vi "ErrorLog_ClearErrors.vi"(7 "Owner":string, 8 "error in (no error)":errorcluster, 11 "reference in":refnum<class "ErrorLog.lvclass">) -> (0 "error out":errorcluster, 3 "reference out":refnum<class "ErrorLog.lvclass">)   [LabVIEW 2014, in "ErrorLog.lvclass"]
uses:
  ErrorLog.lvclass
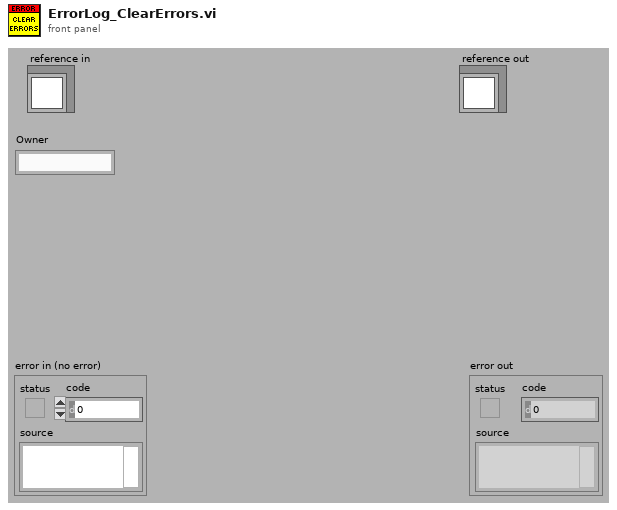
[diagram p1: front panel]
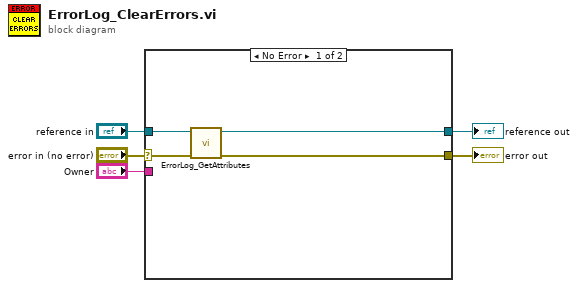
[diagram p0: block diagram]
diagram:
  n1 = case shown="No Error" "error in (no error)" {
    selector: "error in (no error)" -> [w8 w11]
    tunnel: [w6 w11] -> w4
    tunnel: [w7 w10] -> w2
    tunnel: "reference in" -> [w9 w10]
    tunnel: "Owner" -> [_ _]
    frame No Error {
      n2 = call "ErrorLog_GetAttributes.vi"("error in (no error)"=w8, "reference in"=w9) -> ("error out"=w6:errorcluster, "reference out"=w7:refnum<class "ErrorLog.lvclass">)  [unwired: 6 in, 2 out]
    }
    frame Error {
    }
  }
  "error out" <- w4
  "reference out" <- w2
